vi "Callback_SR.vi"(4 "Spoken text box":refnum<vi>, 5 "Event Data":cluster{"sender":refnum<k24>, "e":refnum<k24>}, 6 "Control Ref":refnum<k24>, 7 "Event Common Data":T1) -> ()   [LabVIEW 2013]
uses:
  System.Speech
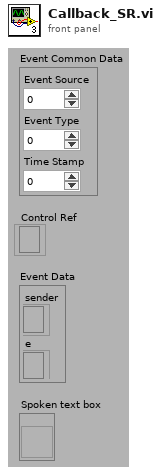
[diagram p1: front panel]
types:
  T1 = cluster{"Event Source":i32, "Event Type":u32, "Time Stamp":u32}
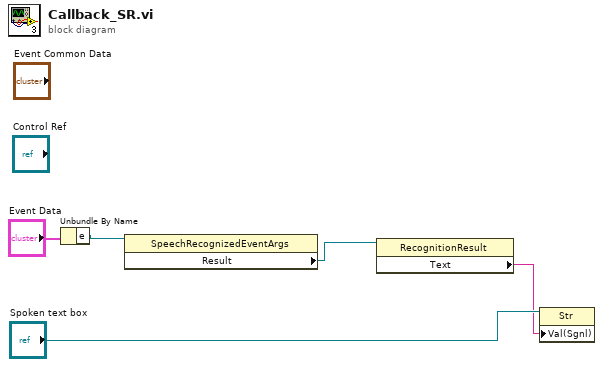
[diagram p0: block diagram]
diagram:
  n1 = Unbundle By Name("Event Data") -> ("e"=w1:refnum<k24>)
  n2 = property class="SpeechRecognizedEventArgs"(reference=w1) -> ("Result"=w5:refnum<k24>)  [unwired: 1 in, 2 out]
  n3 = property class="RecognitionResult"(reference=w5) -> ("Text"=w3:string)  [unwired: 1 in, 2 out]
  n4 = property class="Str"(reference="Spoken text box", "Val(Sgnl)"=w3) -> ()  [unwired: 1 in, 2 out]
